vi "K-Means clustering.vi"(0 "Array":dbl[][](array[numeric])) -> (1 "Mean 1":dbl, 2 "Mean 2":dbl)   [LabVIEW 2013]
uses:
  <vilib>/addons/Machine Learning/NILabs_MLT.lvlib
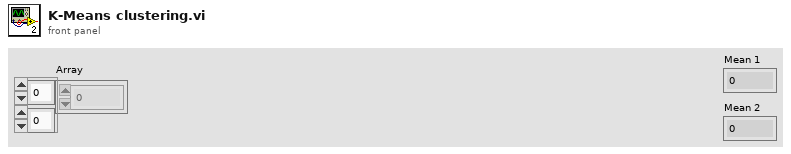
[diagram p1: front panel]
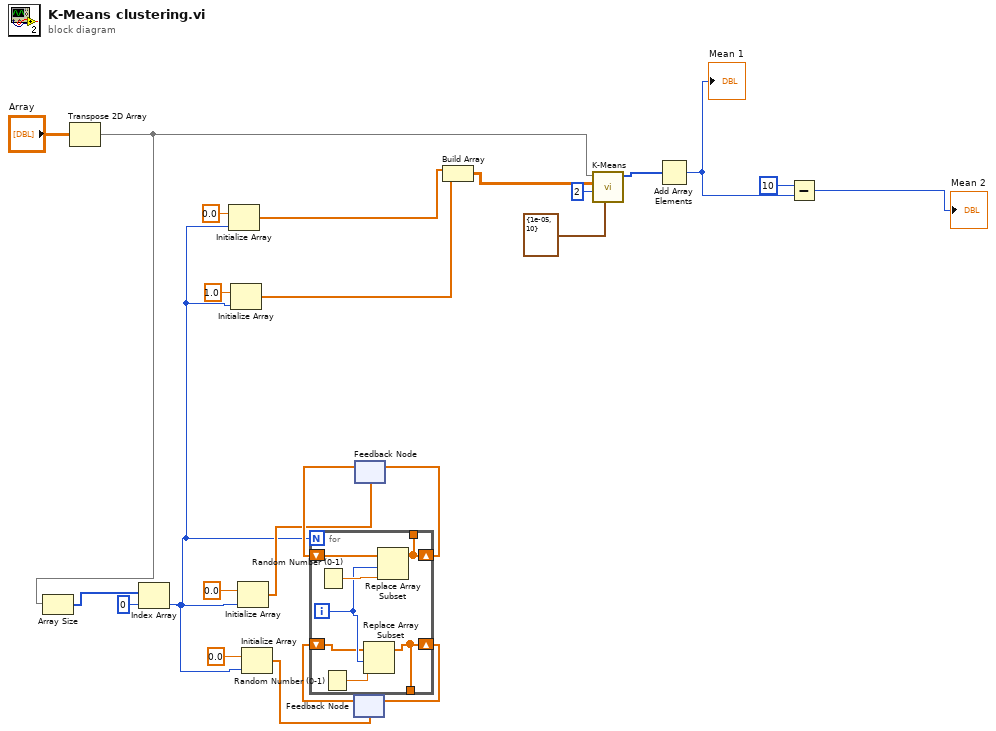
[diagram p0: block diagram]
diagram:
  n1 = Transpose 2D Array(2D array="Array") -> (transposed array=w6:dbl[][])
  n2 = Array Size(array=w6) -> (size(s)=w24:i32[])
  n3 = Index Array(array=w24, index=0) -> (element=w5:i32)
  n4 = Initialize Array(0.0 ("element"), w5) -> (w2:dbl[])
  n5 = Initialize Array(1.0 ("element"), w5) -> (w1:dbl[])
  n6 = Initialize Array(0.0 ("element"), w5) -> (w13:dbl[])
  n7 = Initialize Array(0.0 ("element"), w5) -> (w12:dbl[])
  n8 = feedback #1(w12) -> (w16:dbl[])
  n9 = feedback #2(w13) -> (w14:dbl[])
  n10 = for {
    N: w5 -> [_]
    shift-right: [w25] -> w15
    shift-left: w14 -> [w28]
    shift-right: [w26] -> w17
    shift-left: w16 -> [w27]
    tunnel: [w26] -> _
    tunnel: [w25] -> _
    i -> [w29]
    n11 = Random Number (0-1)() -> (number: 0 to 1=w31:dbl)
    n12 = Random Number (0-1)() -> (number: 0 to 1=w30:dbl)
    n13 = Replace Array Subset(array=w27, new element=w30, index=w29) -> (w26:dbl[])
    n14 = Replace Array Subset(array=w28, new element=w31, index=w29) -> (w25:dbl[])
  }
  n15 = feedback-in #1(w17) -> ()
  n16 = feedback-in #2(w15) -> ()
  n17 = Build Array(w2, w1) -> (w10:dbl[][])
  n18 = call <vilib>:"K-Means.vi"("stopping criteria"=cluster{"tolarence":dbl, "max iterations":i32} {"tolarence"=1e-05, "max iterations"=10}, "# of classes"=2, "Centroids (initial)"=w10, "Data samples"=w6) -> ("Class labels"=w7:i32[])  [unwired: 5 in, 2 out]
  n19 = Add Array Elements(numeric array=w7) -> (sum=w20:i32)
  "Mean 1" <- w20
  n20 = Subtract(x=u8 10, y=w20) -> (x-y=→"Mean 2":i32)
